vi "Test Morphology.vi"(8 "error in (no error)":errorcluster, 11 "Test Case In":refnum<class "Image.lvclass">) -> (0 "error out":errorcluster, 3 "Test Case Out":refnum<class "Image.lvclass">)   [LabVIEW 2020, in "g_ar_toolkit.test.lvlib" / "Image.lvclass"]
uses:
  Image.lvclass
  C:/Program Files (x86)/National Instruments/LabVIEW 2020/vi.lib/Astemes/LUnit/Test Case.lvclass
  g_ar_toolkit.common/Image Size (Integer).ctl
  <vilib>/Astemes/LUnit/Test Case.lvclass/Test Case.ctl
  ff8dbaef-6b31-4074-9b8a-3690e2ff7ea5.vi
  g_ar_toolkit.image/New Image (Greyscale Array).vi
  g_ar_toolkit.image/Get Morphology Structuring Element (Rectangle).vi
  g_ar_toolkit.image/New Image (Greyscale).vi
  g_ar_toolkit.image/Morphology (Erode).vi
  g_ar_toolkit.image/Morphology (Dilate).vi
  g_ar_toolkit.image/Draw Image to Picture (Greyscale).vi
  500a0bd8-6df3-418a-afdb-164a7808fe68.vi
  g_ar_toolkit.image/MorphStructuringElementCore.vi
  g_ar_toolkit.image/New Image (Greyscale).vi/6598b9e0-8a08-46f5-91fd-ca1b87217137.vi
  g_ar_toolkit.image/MorphologyCore.vi
  g_ar_toolkit.image/Draw Image to Picture (Greyscale).vi/9ae995ca-ccda-485c-89ac-02736fde3e8e.vi
  <vilib>/Astemes/LUnit/Append Pass Result.vi
  <vilib>/Astemes/LUnit/Append Fail Result.vi
  <vilib>/Astemes/LUnit/Describe Comparison.vi
  500a0bd8-6df3-418a-afdb-164a7808fe68.vi/9c5d11cd-9439-4240-a1ee-d9baace9c924.vi
  <vilib>/Astemes/LUnit/Run In UI.vi
  <vilib>/Utility/error.llb/Clear Errors.vi
  g_ar_toolkit.common/Module Path.vi
  <vilib>/Utility/error.llb/Error Cluster From Error Code.vi
  <vilib>/Astemes/LUnit/Describe Variant.vi
  Image.lvclass/Image.ctl
  g_ar_toolkit.image/g_ar_toolkit.image.lvlib
  g_ar_toolkit.common/g_ar_toolkit.common.lvlib
  g_ar_toolkit.image/Morphology (Gradient).vi
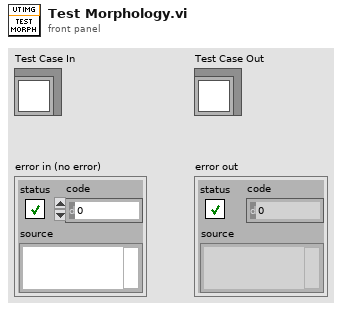
[diagram p1: front panel]
types:
  T1 = typedef "g_ar_toolkit.common.lvlib/Image Size (Integer).ctl" = cluster{"Width":u16, "Height":u16}
  T2 = typedef "g_ar_toolkit.image.lvlib/Greyscale Image.ctl" = refnum<data-value>
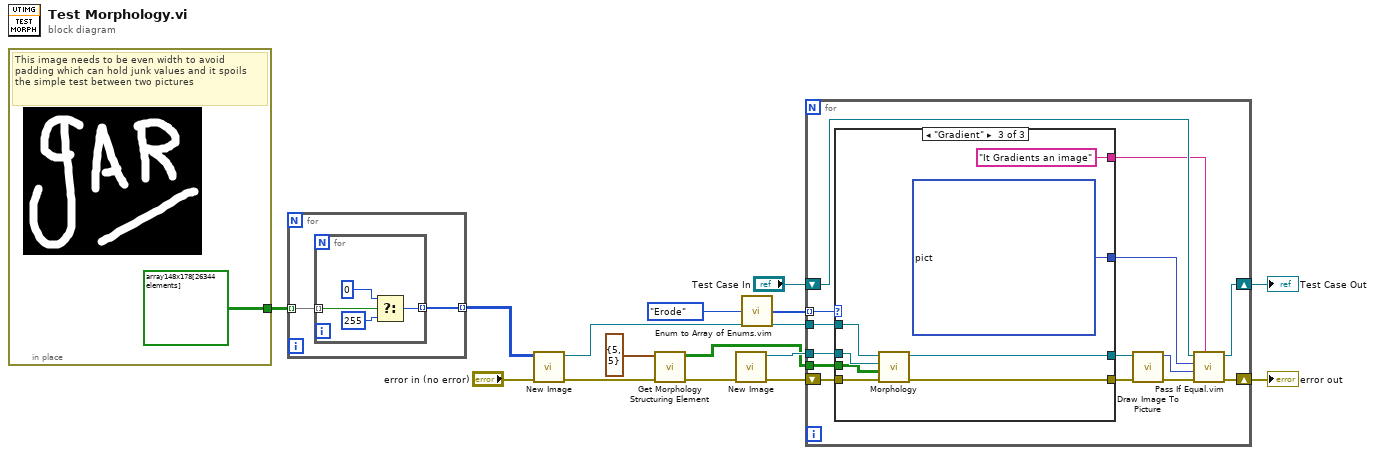
[diagram p0: block diagram]
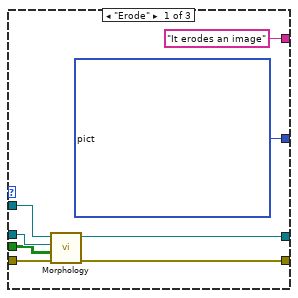
[diagram p2: hidden frame]
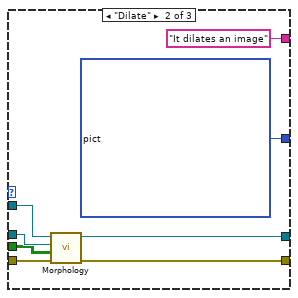
[diagram p3: hidden frame]
diagram:
  n1 = in-place {
    in-place-border: [bool[][] array148x178[26344 elements] ("1-bit pixmap")] -> w15
    # "This image needs to be even width to avoid padding which can hold junk values and it spoils the simple test between two pictures"
  }
  n2 = for {
    tunnel: w15 -> [w18] mode=indexing
    tunnel: [w17] -> w14 mode=indexing
    n3 = for {
      tunnel: w18 -> [w22] mode=indexing
      tunnel: [w20] -> w17 mode=indexing
      n4 = Select(t=u8 0, s=w22, f=u8 255) -> (s? t:f=w20:u8)
    }
  }
  n5 = call-poly "New Image.vi"("error in (no error)"="error in (no error)", "Greyscale Pixels (Default: Empty)"=w14) -> ("error out"=w9:errorcluster, "Greyscale Image"=w13:T2)  [unwired: 8 in]
  n6 = call-poly "Get Morphology Structuring Element.vi"("error in (no error)"=w9, "Size"=T1 {"Width"=5, "Height"=5}) -> ("error out"=w8:errorcluster, "Structuring Element"=w11:bool[][])  [unwired: 8 in]
  n7 = call-poly "New Image.vi"("error in (no error)"=w8) -> ("error out"=w7:errorcluster, "New Greyscale Image"=w12:T2)  [unwired: 9 in]
  n8 = call "Enum to Array of Enums.vim"("enum"=enum16{"Erode", "Dilate", "Gradient"}."Erode") -> ("array of enums"=w1:enum16{"Erode", "Dilate", "Gradient"}[])
  n9 = for {
    tunnel: w13 -> [w36]
    tunnel: w12 -> [w35]
    tunnel: w11 -> [w34]
    shift-right: [w29] -> w6
    shift-left: w7 -> [w33]
    shift-right: [w27] -> w3
    shift-left: "Test Case In" -> [w28]
    tunnel: w1 -> [w24] mode=indexing
    n10 = case shown="\"Gradient\"" w24 {
      tunnel: w36 -> [w44 w52 w60]
      tunnel: w35 -> [w43 w51 w59]
      tunnel: w34 -> [w42 w50 w58]
      tunnel: w33 -> [w41 w49 w57]
      tunnel: [w40 w48 w56] -> w32
      tunnel: [w39 w47 w55] -> w31
      tunnel: ["It erodes an image" ("Description") "It dilates an image" ("Description") "It Gradients an image" ("Description")] -> w26
      tunnel: [picture bytes[28424] ("Picture") picture bytes[28424] ("Picture") picture bytes[28424] ("Picture")] -> w25
      frame "Erode" {
        n11 = call-poly "Morphology.vi"("error in (no error)"=w41, "Structuring Element"=w42, "Morphology Result"=w43, "Greyscale Image-Source"=w44) -> ("error out"=w39:errorcluster, "Morphology Result (Duplicate)"=w40:T2)  [unwired: 6 in]
      }
      frame "Dilate" {
        n12 = call-poly "Morphology.vi"("error in (no error)"=w49, "Structuring Element"=w50, "Morphology Result"=w51, "Greyscale Image-Source"=w52) -> ("error out"=w47:errorcluster, "Morphology Result (Duplicate)"=w48:T2)  [unwired: 6 in]
      }
      frame "Gradient" {
        n13 = call-poly "Morphology.vi"("error in (no error)"=w57, "Structuring Element"=w58, "Morphology Result"=w59, "Greyscale Image-Source"=w60) -> ("error out"=w55:errorcluster, "Morphology Result (Duplicate)"=w56:T2)  [unwired: 6 in]
      }
    }
    n14 = call-poly "Draw Image To Picture.vi"("error in (no error)"=w31, "Greyscale Image Source"=w32) -> ("error out"=w30:errorcluster, "Picture"=w23:picture)  [unwired: 8 in]
    n15 = call "Pass If Equal.vim"("Description"=w26, "error in (no error)"=w30, "Actual"=w23, "Expected"=w25, "LUnit Test Case In"=w28) -> ("error out"=w29:errorcluster, "LUnit Test Case Out"=w27:refnum<class "Image.lvclass">)  [unwired: 5 in]
  }
  "error out" <- w6
  "Test Case Out" <- w3
